vi "motor test.vi"() -> ()   [LabVIEW 2025]
uses:
  Classes/Stepper/Stepper.lvclass
  <vilib>/Handler Framework/CmdQueue/Enqueue Single.vi
  <vilib>/Handler Framework/Handler Framework.lvlib
panel:
  in  "Clear error":bool
  out "error out":errorcluster
  in  "Tab Control":enum32{"Check Parameters", "Write Parameters"}(tab)
  in  "Parameters":u32[](array[numeric]) format="%.0x"
  out "Hex Result":u32[](array[numeric]) format="%.0x"
  out "Decimal Result":u32[](array[numeric])
  in  "Check Params":bool
  out "Bin Result":u32[](array[numeric]) format="%.0b"
  in  "Parameters to Write":u32[](array[numeric]) format="%.0x"
  # "ERRORS:"
  # "CHECK PARAMETERS:"
  # "WRITE PARAMETERS:"
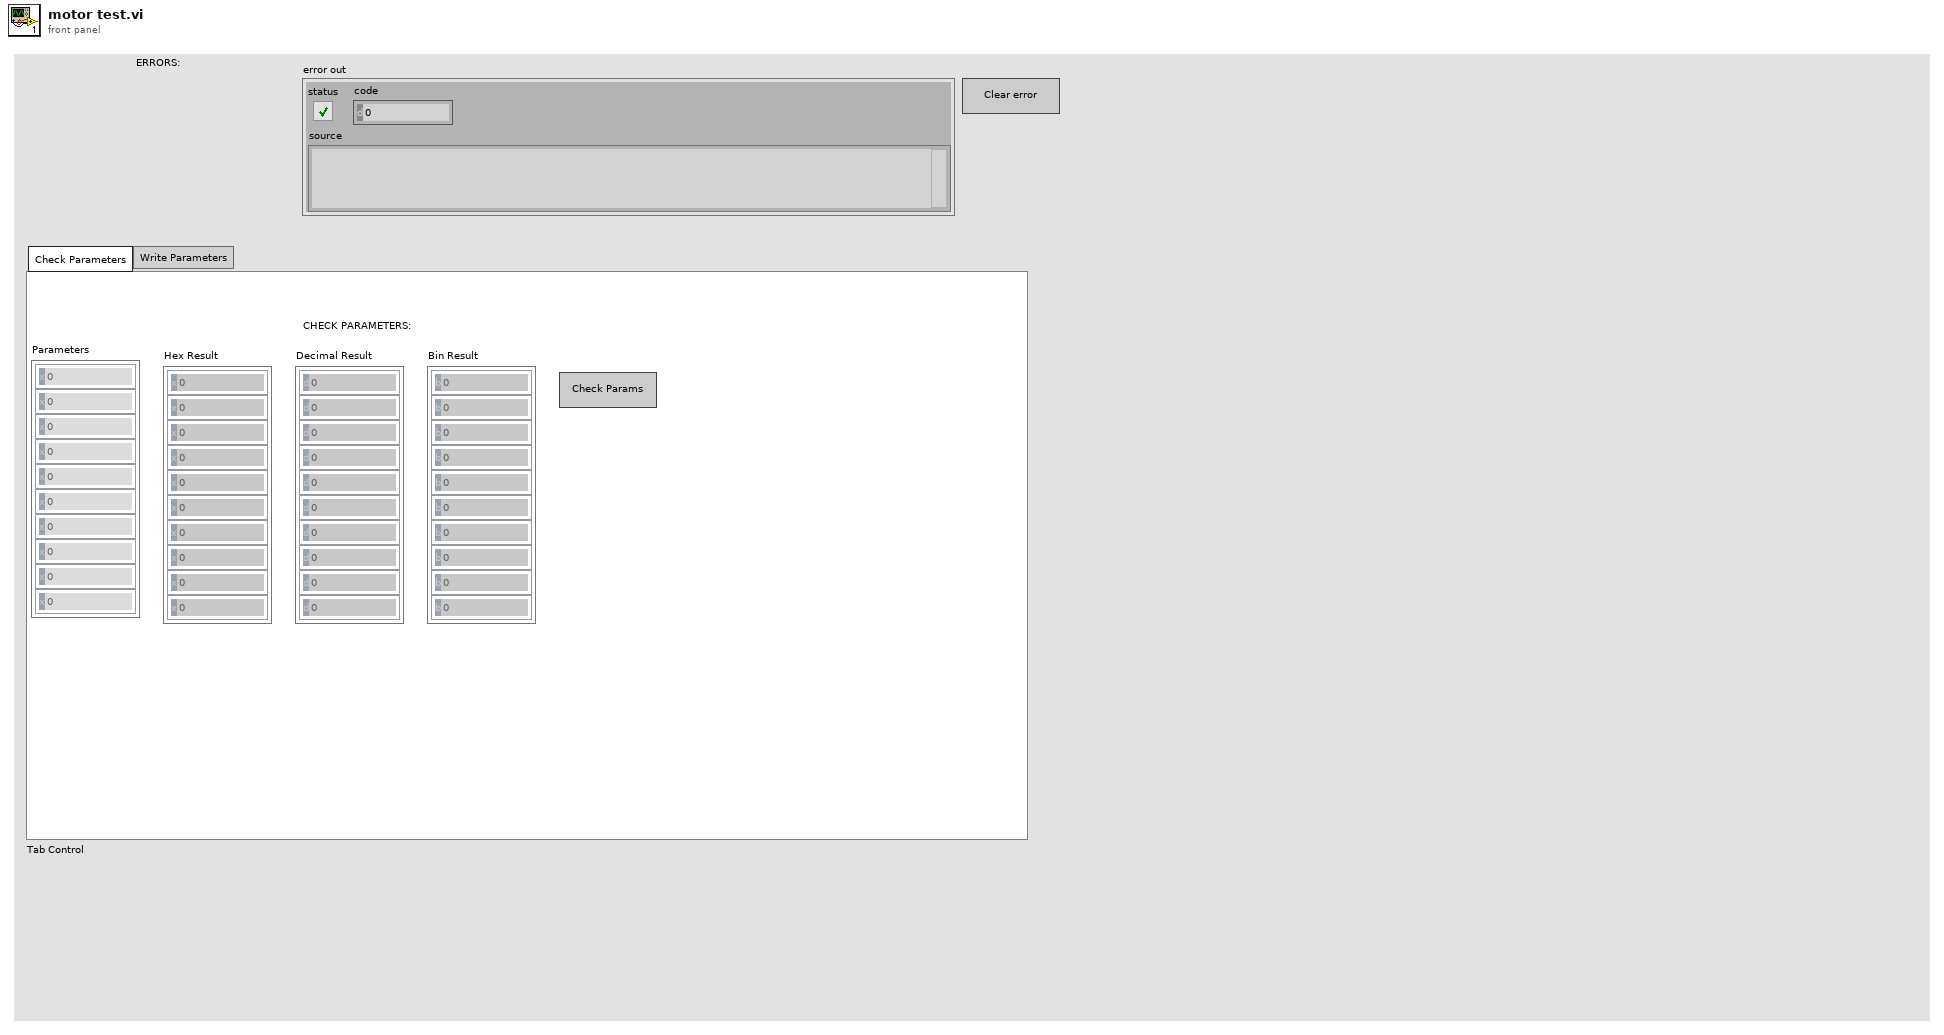
[diagram p1: front panel]
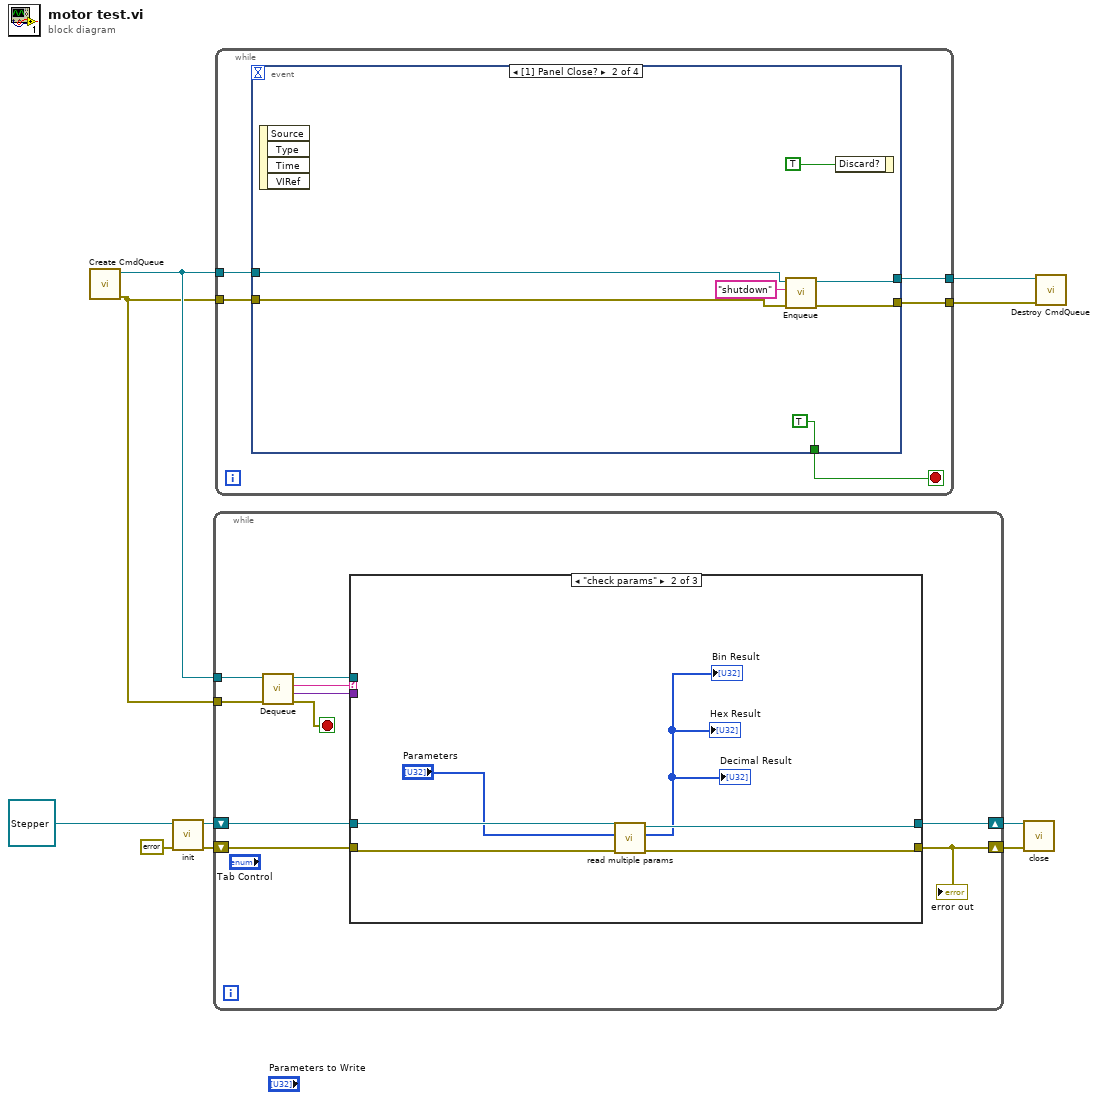
[diagram p0: block diagram]
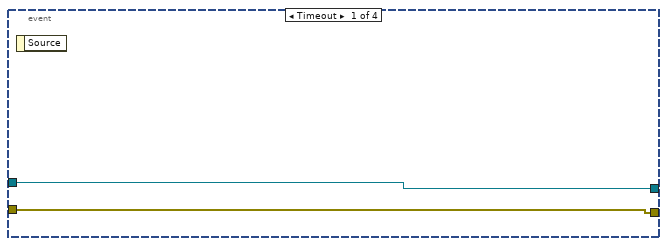
[diagram p4: hidden frame]
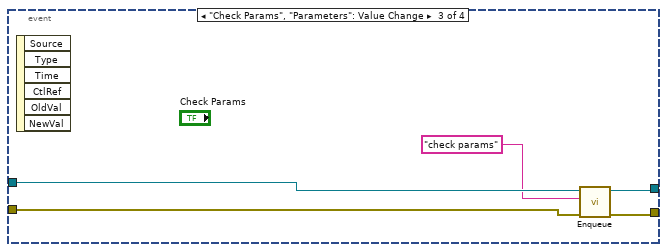
[diagram p5: hidden frame]
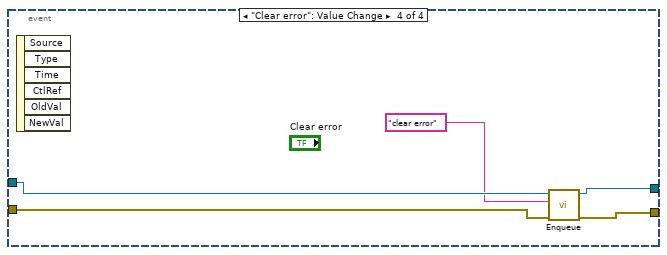
[diagram p6: hidden frame]
diagram:
  n1 = call <vilib>:"Create CmdQueue.vi"() -> ("error out"=w7:errorcluster, "CmdQueue out"=w10:refnum<queue>)  [unwired: 10 in]
  n2 = call-dynamic "init.vi"("error in (no error)"=errorcluster {"status"=FALSE, "code"=0, "source"=""}, "Stepper in"=refnum<class "Stepper.lvclass"> refnum ("Stepper.lvclass")) -> ("error out"=w5:errorcluster, "Stepper out"=w6:refnum<class "Stepper.lvclass">)  [unwired: 8 in]
  n3 = while {
    tunnel: w10 -> [w20]
    tunnel: w7 -> [w19]
    shift-right: [w12] -> w4
    shift-left: w5 -> [w13]
    shift-right: [w11] -> w3
    shift-left: w6 -> [w14]
    stop <- w16 stop-if-true
    n4 = call <vilib>:"Dequeue.vi"("error in (no error)"=w19, "CmdQueue in"=w20) -> ("error out"=w16:errorcluster, "value"=w17:variant, "cmd"=w18:string, "CmdQueue out"=w15:refnum<queue>)  [unwired: 5 in, 1 out]
    n5 = case shown="\"check params\"" w18 {
      tunnel: w17 -> [_ _ _]
      tunnel: w15 -> [_ _ _]
      tunnel: w14 -> [w21 w28 w29]
      tunnel: w13 -> [w22 w24 _]
      tunnel: [w22 w25 _] -> w12
      tunnel: [w21 w26 w29] -> w11
      frame "", Default {
      }
      frame "check params" {
        n6 = call-dynamic "read multiple params.vi"("error in (no error)"=w24, "Parameters"="Parameters", "Stepper in"=w28) -> ("error out"=w25:errorcluster, "Hex Result"=→"Hex Result" →"Decimal Result" →"Bin Result":u32[], "Stepper out"=w26:refnum<class "Stepper.lvclass">)  [unwired: 6 in]
      }
      frame "clear error" {
      }
    }
    "error out" <- w12
  }
  n7 = while {
    tunnel: w10 -> [w34]
    tunnel: [w33] -> w9
    tunnel: [w32] -> w8
    tunnel: w7 -> [w31]
    stop <- w30 stop-if-true
    n8 = event shown="[1] Panel Close?" {
      selector: _ -> [_ _ _ _]
      dyn-events: _ -> [_ _ _ _]
      timeout: _ -> [_ _ _ _]
      tunnel: w34 -> [w36 w39 w46 w51]
      tunnel: [w36 w41 w48 w53] -> w33
      tunnel: [w35 w40 w47 w52] -> w32
      tunnel: w31 -> [w35 w38 w45 w50]
      tunnel: [_ TRUE _ _] -> w30
      event Timeout {
        n9 = event-data() -> ()  [unwired: 1 in, 1 out]
      }
      event Panel Close? {
        n10 = event-data() -> ()  [unwired: 1 in, 4 out]
        n11 = call-poly <vilib>:"Enqueue.vi"("error in (no error)"=w38, "Command"="shutdown", "CmdQueue in"=w39) -> ("error out"=w40:errorcluster, "CmdQueue out"=w41:refnum<queue>)  [unwired: 7 in]
        n12 = event-data("Discard?"=TRUE) -> ()  [unwired: 1 in, 1 out]
      }
      event "Check Params", "Parameters": Value Change {
        n13 = event-data() -> ()  [unwired: 1 in, 6 out]
        n14 = call-poly <vilib>:"Enqueue.vi"("error in (no error)"=w45, "Command"="check params", "CmdQueue in"=w46) -> ("error out"=w47:errorcluster, "CmdQueue out"=w48:refnum<queue>)  [unwired: 7 in]
      }
      event "Clear error": Value Change {
        n15 = event-data() -> ()  [unwired: 1 in, 6 out]
        n16 = call-poly <vilib>:"Enqueue.vi"("error in (no error)"=w50, "Command"="clear error", "CmdQueue in"=w51) -> ("error out"=w52:errorcluster, "CmdQueue out"=w53:refnum<queue>)  [unwired: 7 in]
      }
    }
  }
  n17 = call-dynamic "close.vi"("error in (no error)"=w4, "Stepper in"=w3) -> ()  [unwired: 8 in, 2 out]
  n18 = call <vilib>:"Destroy CmdQueue.vi"("error in (no error)"=w8, "CmdQueue in"=w9) -> ()  [unwired: 9 in, 1 out]
